vi "SI_avg_Loop_n.vi"(0 "SIClass in":refnum<class "SIClass.lvclass">, 5 "Loop ID":enum16{"10", "20", "30", "40"}(ring), 7 "3 JECxx CT001A XQ01":dbl, 9 "3 JECxx CT001B XQ01":dbl, 11 "error in (no error)":errorcluster) -> (4 "SIClass out":refnum<class "SIClass.lvclass">, 8 "Numeric":dbl, 15 "error out":errorcluster)   [LabVIEW 2022 SP3, in "SIClass.lvclass"]
uses:
  SIClass.lvclass
  SIClass.lvclass/SIClass.ctl
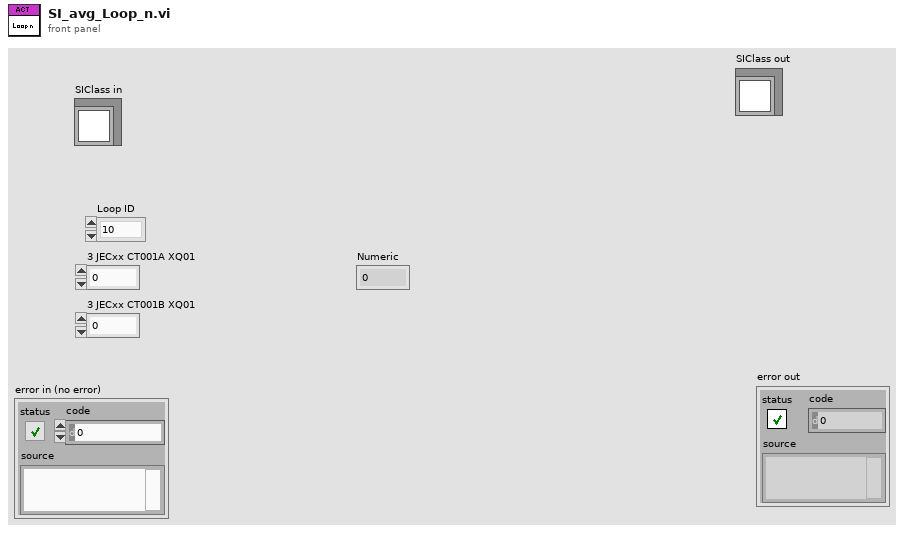
[diagram p1: front panel]
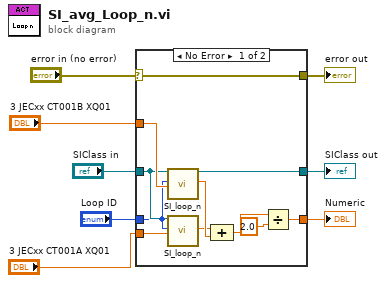
[diagram p0: block diagram]
diagram:
  n1 = case shown="No Error" "error in (no error)" {
    selector: "error in (no error)" -> [w13 _]
    tunnel: "3 JECxx CT001A XQ01" -> [w15 _]
    tunnel: "3 JECxx CT001B XQ01" -> [w14 _]
    tunnel: [w13 _] -> w5
    tunnel: [w12 _] -> w4
    tunnel: "SIClass in" -> [w11 _]
    tunnel: [w10 _] -> w2
    tunnel: "Loop ID" -> [w9 _]
    frame No Error {
      n2 = call-dynamic "SI_loop_n.vi"("SIClass in"=w11, "Loop ID"=w9, "Input"=w14) -> ("SIClass out"=w10:refnum<class "SIClass.lvclass">, "Output"=w17:dbl)  [unwired: 14 in, 1 out]
      n3 = call-dynamic "SI_loop_n.vi"("SIClass in"=w11, "Loop ID"=w9, "Input"=w15) -> ("Output"=w16:dbl)  [unwired: 14 in, 2 out]
      n4 = Compound Arithmetic op=ADD(w16, w17) -> (w18:dbl)
      n5 = Divide(x=w18, y=2.0) -> (x/y=w12:dbl)
    }
    frame Error {
    }
  }
  "error out" <- w5
  "Numeric" <- w4
  "SIClass out" <- w2
